vi "Traverse-Settings-Selector.vi"() -> ()   [LabVIEW 2017]
uses:
  TypeDefs/Traverse-Types-TD.ctl
  Settings/Settings-Control.ctl
  TypeDefs/Position-Info-TD.ctl
  Settings/Traverse-Settings-Global.vi
  Globals/Trav-Positon-Info.vi
panel:
  in  "Position Info IN":T1
  in  "Settings":T2
  in  "Traverse":T3 items=["Strut", "Wind Tunnel"]
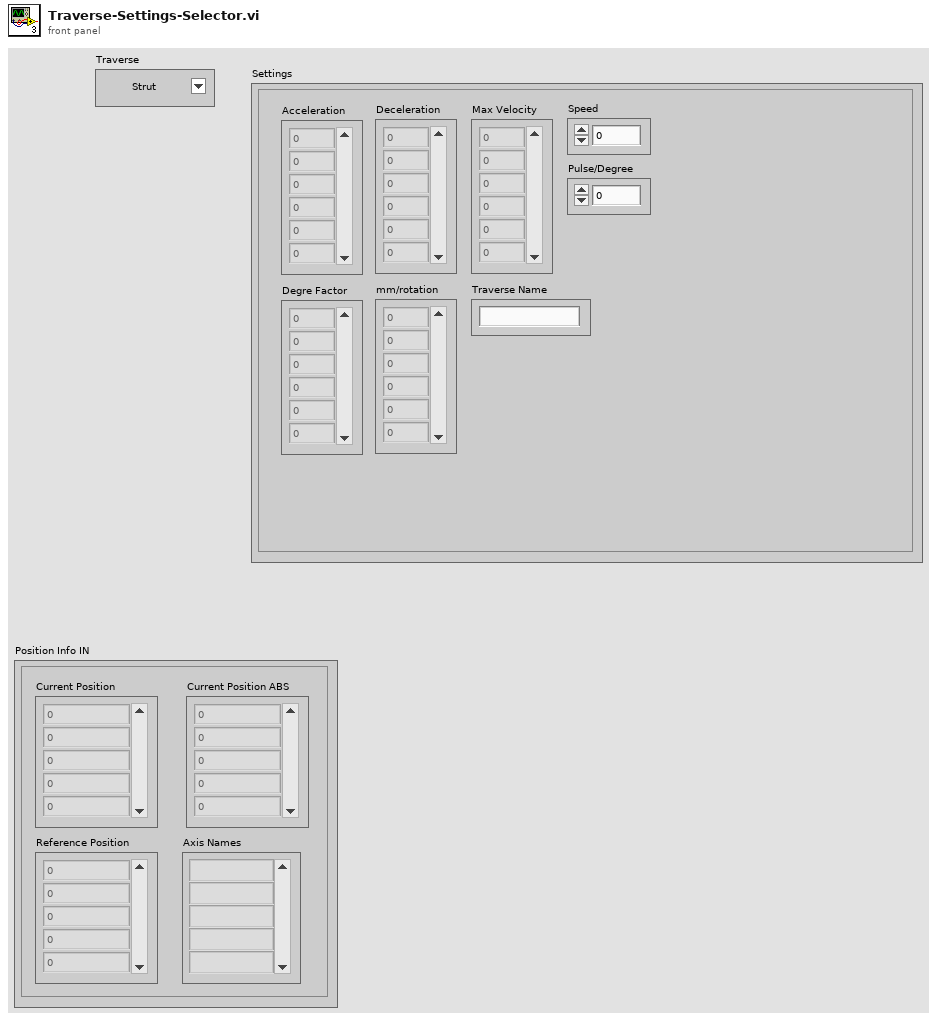
[diagram p1: front panel]
types:
  T1 = typedef "Position-Info-TD.ctl" = cluster{"Current Position ABS":dbl[], "Current Position":dbl[], "Reference Position":dbl[], "Axis Names":string[]}
  T2 = typedef "Settings-Control.ctl" = cluster{"Acceleration":dbl[], "Deceleration":dbl[], "Max Velocity":dbl[], "Speed":dbl, "Pulse/Degree":dbl, "Degre Factor":dbl[], "mm/rotation":dbl[], "Traverse Name":string}
  T3 = typedef "Traverse-Types-TD.ctl" = u16
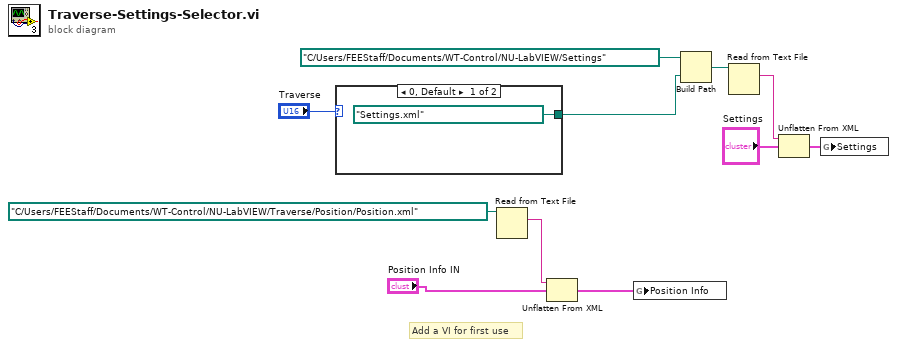
[diagram p0: block diagram]
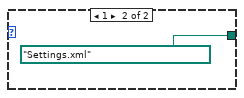
[diagram p2: hidden frame]
diagram:
  # "Add a VI for first use"
  n1 = case shown="0, Default" "Traverse" {
    tunnel: [path "Settings.xml" ("File Path Control") path "Settings.xml" ("File Path Control")] -> w7
    frame 0, Default {
    }
    frame 1 {
    }
  }
  n2 = Read from Text File(file (use dialog)=path "C:/Users/FEEStaff/Documents/WT-Control/NU-LabVIEW/Traverse/Position/Position.xml") -> (text=w4:string)  [unwired: 3 in, 3 out]
  n3 = Unflatten From XML(xml string=w4, type="Position Info IN") -> (value=w2:T1)  [unwired: 1 in, 1 out]
  n4 = global write "Trav-Positon-Info.vi" "Position Info"(w2) -> ()
  n5 = Build Path(base path=path "C:/Users/FEEStaff/Documents/WT-Control/NU-LabVIEW/Settings" ("Settings Location"), name or relative path=w7) -> (appended path=w6:path)
  n6 = Read from Text File(file (use dialog)=w6) -> (text=w8:string)  [unwired: 3 in, 3 out]
  n7 = Unflatten From XML(xml string=w8, type="Settings") -> (value=w9:T2)  [unwired: 1 in, 1 out]
  n8 = global write "Traverse-Settings-Global.vi" "Settings"(w9) -> ()
